vi "Set LakeShore 340 Set Point.vi"(7 "Set point":dbl format="%.2f", 8 "error in (no error)":errorcluster, 10 "Output #":i32=1, 11 "VISA Resource Name":refnum<visa-resource-name>) -> (0 "error out":errorcluster, 3 "VISA Resource Name Out":refnum<visa-resource-name>)   [LabVIEW 2024]
uses:
  Simple VISA Reader/Simple VISA Reader Driver.lvclass
  GPIB/VISA  Send Receive.vi
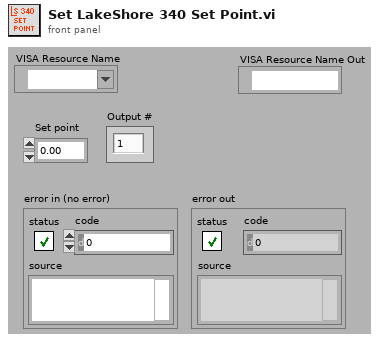
[diagram p1: front panel]
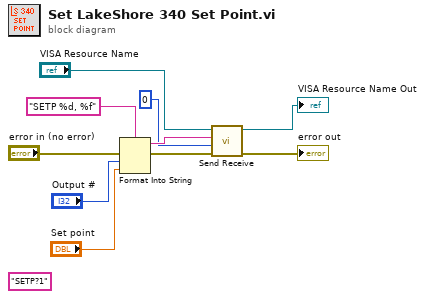
[diagram p0: block diagram]
diagram:
  (unwired) "SETP?1" ("data string")
  n1 = Format Into String(format string="SETP %d, %f" ("write buffer"), error in="error in (no error)", "Output #", "Set point") -> (resulting string=w2:string, error out=w4:errorcluster)  [unwired: 1 in]
  n2 = call-poly "Send Receive.vi"("error in (no error)"=w4, "Receive count"=0, "data string in"=w2, "VISA Resource Name"="VISA Resource Name") -> ("error out"=→"error out":errorcluster, "VISA Resource Name Out"=→"VISA Resource Name Out":refnum<visa-resource-name>)  [unwired: 5 in, 1 out]
